vi "SupportAttackerRole.vi"(8 "error in (no error)":errorcluster, 11 "SupportAttackerRole in":refnum<class "SupportAttackerRole.lvclass">) -> (0 "error out":errorcluster, 3 "SupportAttackerRole out":refnum<class "SupportAttackerRole.lvclass">)   [LabVIEW 2023, in "SupportAttackerRole.lvclass"]
uses:
  SupportAttackerRole.lvclass
  C:/Users/ebert/Documents/codes/SSL/repo/SSL_AI/Role_class/Role.lvclass
  Robot_class/Robot.lvclass
  Game_class/Game.lvclass
  Role_class/Role.lvclass/Role.ctl
  SupportAttackerRole_states.ctl
  STP_Parameters/TestSkills.ctl
  Tacticbook_class/Tacticbook.lvclass/Tacticbook.ctl
  Tacticbook_class/Read TestTactic.vi
  Role_class/Read Tacticbook.vi
  Role_class/Write Tacticbook.vi
  Role_class/Write tactic_index.vi
  Role_class/Read RobotRef.vi
  Tacticbook_class/Tacticbook.lvclass
  TestTactic_class/TestTactic.lvclass
panel:
  in  "Game in":refnum<class "Game.lvclass">
  out "Robot out":refnum<class "Robot.lvclass">
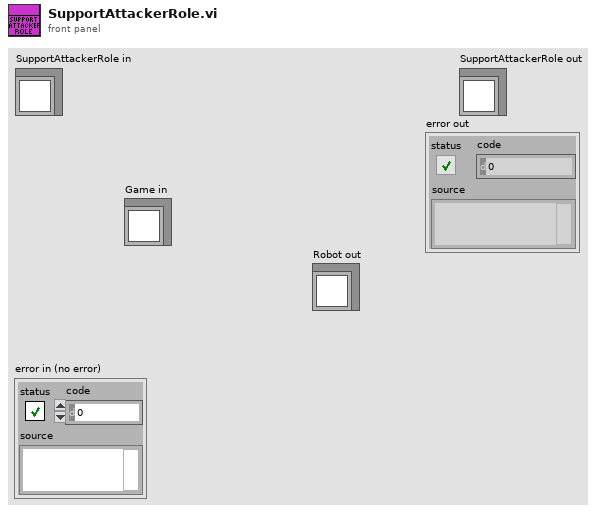
[diagram p1: front panel]
types:
  T1 = typedef "SupportAttackerRole.lvclass/SupportAttackerRole_states.ctl" = enum16{"Position", "WaitPass", "Exit"}
  T2 = typedef "TestSkills.ctl" = enum16{"CirculateBall", "ProtectBall", "ReceivePass", "GoTo"}
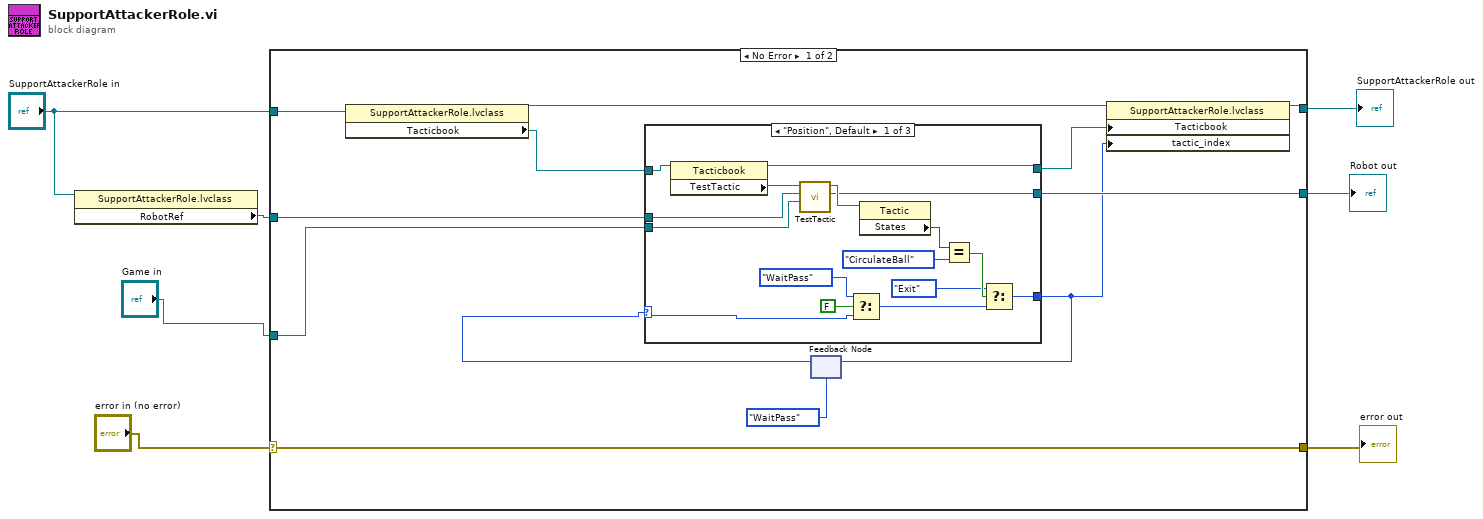
[diagram p0: block diagram]
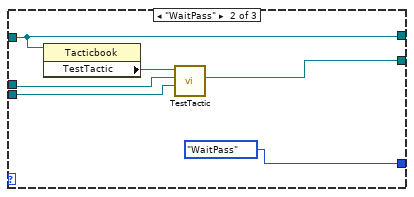
[diagram p2: hidden frame]
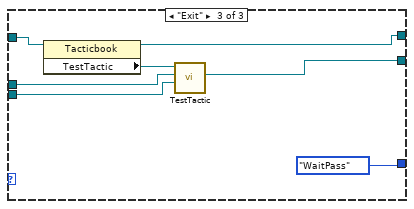
[diagram p3: hidden frame]
diagram:
  n1 = property class="SupportAttackerRole.lvclass"(reference="SupportAttackerRole in") -> ("RobotRef"=w5:refnum<class "Robot.lvclass">)  [unwired: 1 in, 2 out]
  n2 = case shown="No Error" "error in (no error)" {
    selector: "error in (no error)" -> [w19 w51]
    tunnel: [w19 w51] -> w1
    tunnel: [w18 w49] -> w3
    tunnel: w5 -> [w13 w50]
    tunnel: [w15 w50] -> w7
    tunnel: "Game in" -> [w8 _]
    tunnel: "SupportAttackerRole in" -> [w9 w49]
    frame No Error {
      n3 = property class="SupportAttackerRole.lvclass"(reference=w9) -> (reference out=w17:refnum<class "SupportAttackerRole.lvclass">, "Tacticbook"=w16:refnum<class "Tacticbook.lvclass">)  [unwired: 1 in, 1 out]
      n4 = feedback #1(SupportAttackerRole_states."WaitPass" ("States")) -> (w10:T1)
      n5 = case shown="\"Position\", Default" w10 {
        selector: w10 -> [w26 _ _]
        tunnel: [w25 SupportAttackerRole_states."WaitPass" ("States") SupportAttackerRole_states."WaitPass" ("States")] -> w12
        tunnel: w16 -> [w22 w41 w47]
        tunnel: w13 -> [w21 w39 w46]
        tunnel: [w24 w37 w44] -> w15
        tunnel: [w23 w41 w43] -> w14
        tunnel: w8 -> [w20 w38 w45]
        frame "Position", Default {
          n6 = property class="Tacticbook"(reference=w22) -> (reference out=w23:refnum<class "Tacticbook.lvclass">, "TestTactic"=w31:refnum<class "TestTactic.lvclass">)  [unwired: 1 in, 1 out]
          n7 = call-dynamic "TestTactic.vi"("Game in"=w20, "Robot"=w21, "Tactic in"=w31) -> ("Robot out"=w24:refnum<class "Robot.lvclass">, "Tactic out"=w30:refnum<class "TestTactic.lvclass">)  [unwired: 6 in, 1 out]
          n8 = Select(t=SupportAttackerRole_states."WaitPass" ("States"), s=FALSE, f=w26) -> (s? t:f=w33:T1)
          n9 = property class="Tactic"(reference=w30) -> ("States"=w34:T2)  [unwired: 1 in, 2 out]
          n10 = Equal?(x=w34, y=TestSkills."CirculateBall") -> (x = y?=w35:bool)
          n11 = Select(t=SupportAttackerRole_states."Exit" ("States"), s=w35, f=w33) -> (s? t:f=w25:T1)
        }
        frame "WaitPass" {
          n12 = property class="Tacticbook"(reference=w41) -> ("TestTactic"=w40:refnum<class "TestTactic.lvclass">)  [unwired: 1 in, 2 out]
          n13 = call-dynamic "TestTactic.vi"("Game in"=w38, "Robot"=w39, "Tactic in"=w40) -> ("Robot out"=w37:refnum<class "Robot.lvclass">)  [unwired: 6 in, 2 out]
        }
        frame "Exit" {
          n14 = property class="Tacticbook"(reference=w47) -> (reference out=w43:refnum<class "Tacticbook.lvclass">, "TestTactic"=w48:refnum<class "TestTactic.lvclass">)  [unwired: 1 in, 1 out]
          n15 = call-dynamic "TestTactic.vi"("Game in"=w45, "Robot"=w46, "Tactic in"=w48) -> ("Robot out"=w44:refnum<class "Robot.lvclass">)  [unwired: 6 in, 2 out]
        }
      }
      n16 = feedback-in #1(w12) -> ()
      n17 = property class="SupportAttackerRole.lvclass"(reference=w17, "Tacticbook"=w14, "tactic_index"=w12) -> (reference out=w18:refnum<class "SupportAttackerRole.lvclass">)  [unwired: 1 in, 1 out]
    }
    frame Error {
    }
  }
  "SupportAttackerRole out" <- w3
  "Robot out" <- w7
  "error out" <- w1
